vi "GEN40-38-LAN Verify Device Firmware.vi"(8 "error in":errorcluster, 11 "Revisions":string) -> (0 "error out":errorcluster)   [LabVIEW 2018, in "GEN40-38-LAN.lvlib" / "GEN40-38-LAN.lvclass"]
doc: "This VI is used to inquire for the Power Supply firmware. Only firmware revision ending in 2.1 will work with this class driver."
uses:
  GEN40-38-LAN.lvclass
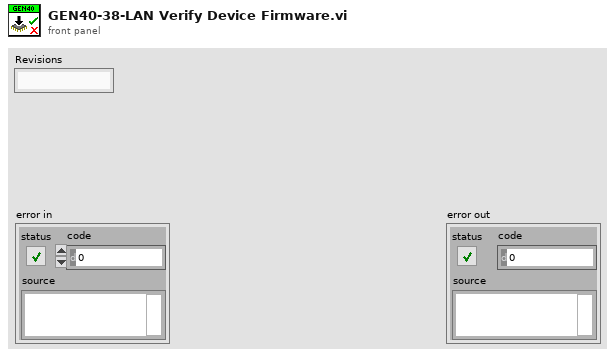
[diagram p1: front panel]
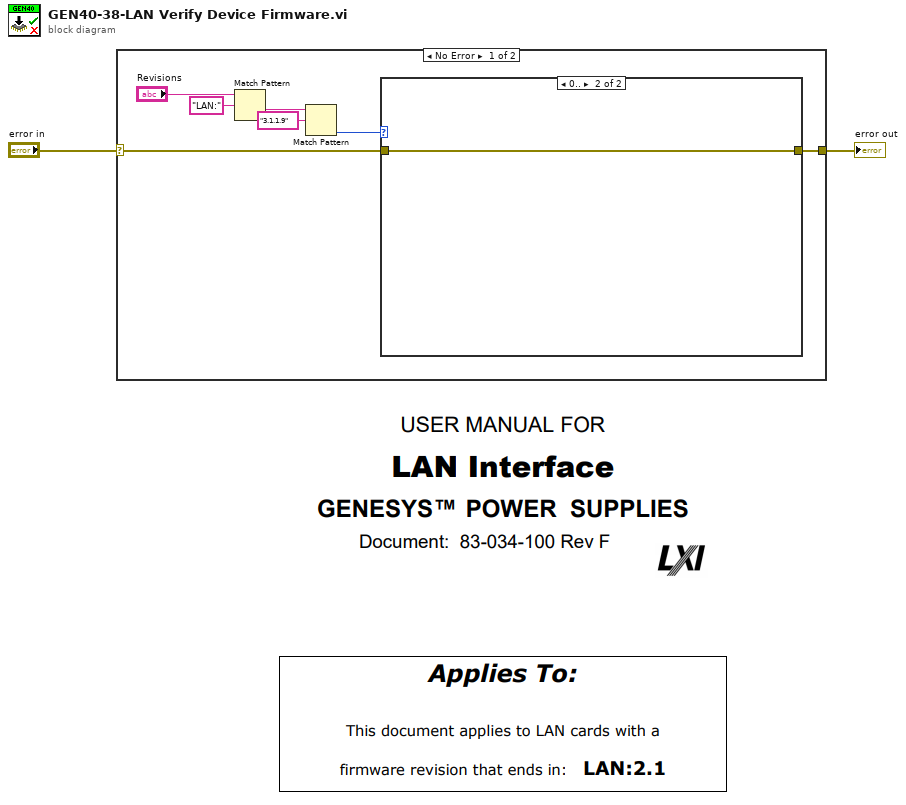
[diagram p0: block diagram]
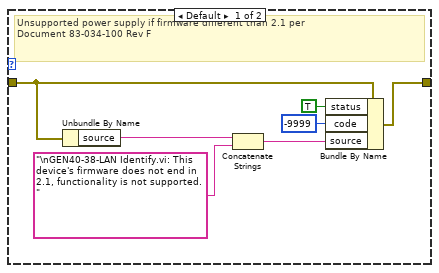
[diagram p2: hidden frame]
diagram:
  n1 = case shown="No Error" "error in" {
    selector: "error in" -> [w4 w18]
    tunnel: [w3 w18] -> w1
    frame No Error {
      n2 = Match Pattern(string="Revisions", regular expression="LAN:") -> (after substring=w8:string)  [unwired: 1 in, 3 out]
      n3 = Match Pattern(string=w8, regular expression="3.1.1.9") -> (offset past match=w6:i32)  [unwired: 1 in, 3 out]
      n4 = case shown="0.." w6 {
        tunnel: [w16 w17] -> w3
        tunnel: w4 -> [w15 w17]
        frame Default {
          # "Unsupported power supply if firmware different than 2.1 per \nDocument 83-034-100 Rev F"
          n5 = Unbundle By Name(w15) -> ("source"=w14:string)
          n6 = Concatenate Strings(w14, "\nGEN40-38-LAN Identify.vi: This device's firmware does not end in 2.1, functionality is not supported.") -> (w13:string)
          n7 = Bundle By Name(cluster=w15, "status"=TRUE, "code"=-9999, "source"=w13) -> (w16:errorcluster)
        }
        frame 0.. {
        }
      }
    }
    frame Error {
    }
  }
  "error out" <- w1
